vi "Create NI-DCPower Sessio.vi"(8 "error in (no error)":errorcluster, 10 "session information":T3, 11 "gRPC channel pool":T1) -> (0 "error out":errorcluster, 2 "instrument handle":refnum<k15>, 3 "gRPC channel pool out":T1)   [LabVIEW 2020, in "NIDCPowerSourceDCVoltage.lvlib"]
doc: "Creates and returns an gRPC based NI DC power instrument handle."
uses:
  NIDCPowerSourceDCVoltage.lvlib
  <vilib>/MeasurementLink/MeasurementLink Session Management Client/RPC Messages/ni_measurementlink_sessionmanagement_v1_SessionInformation.ctl
  <vilib>/MeasurementLink/MeasurementLink Session Management Client/RPC Messages/nidevice_grpc_Session.ctl
  <vilib>/MeasurementLink/MeasurementLink Session Management Client/RPC Messages/ni_measurementlink_sessionmanagement_v1_ChannelMapping.ctl
  GRPC Clients.ctl
  <vilib>/gRPC/LabVIEW gRPC Library/Shared/grpcId.ctl
  <vilib>/MeasurementLink/MeasurementLink Session Management Client/MeasurementLink Session Management Client.lvlib
  <vilib>/gRPC/LabVIEW gRPC Library/grpc-lvsupport-release.lvlib
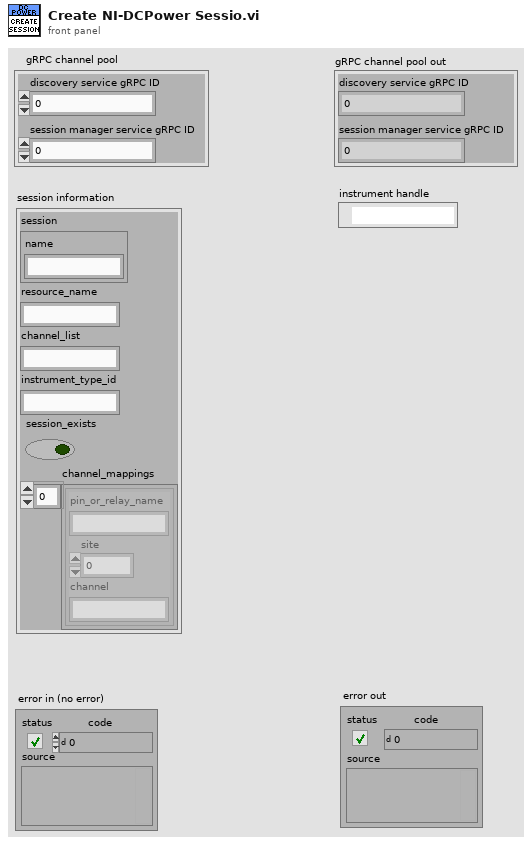
[diagram p1: front panel]
types:
  T1 = typedef "NIDCPowerSourceDCVoltage.lvlib/GRPC Clients.ctl" = cluster{"discovery service gRPC ID":T2, "session manager service gRPC ID":T2}
  T2 = typedef "grpc-lvsupport-release.lvlib/grpcId.ctl" = u64
  T3 = typedef "MeasurementLink Session Management Client.lvlib/ni_measurementlink_sessionmanagement_v1_SessionInformation.ctl" = cluster{"session":T4, "resource_name":string, "channel_list":string, "instrument_type_id":string, "session_exists":bool, "channel_mappings":T5[]}
  T4 = typedef "MeasurementLink Session Management Client.lvlib/nidevice_grpc_Session.ctl" = cluster{"name":string}
  T5 = typedef "MeasurementLink Session Management Client.lvlib/ni_measurementlink_sessionmanagement_v1_ChannelMapping.ctl" = cluster{"pin_or_relay_name":string, "site":i32, "channel":string}
  T6 = typedef "MeasurementLink Discovery Client.lvlib/ni_measurementlink_discovery_v1_ServiceLocation.ctl" = cluster{"location":string, "insecure_port":string, "ssl_authenticated_port":string}
  T7 = typedef "niDCPower gRPC Device Server.ctl" = cluster{"session name":string, "address (localhost)":string, "port (31763)":u32}
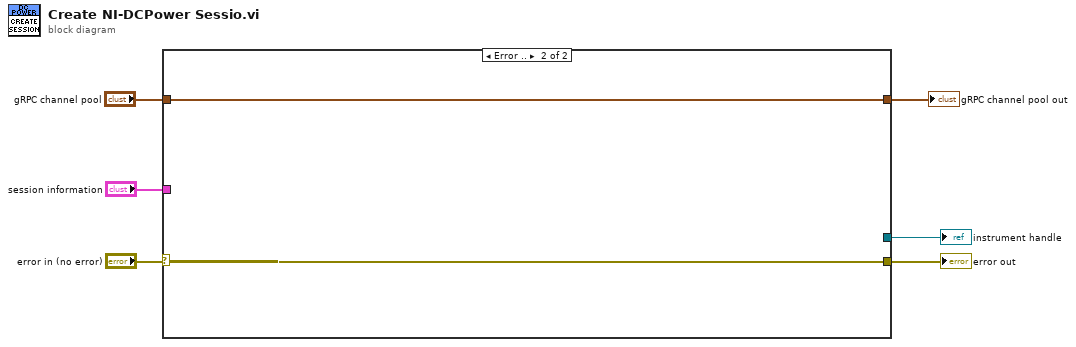
[diagram p0: block diagram]
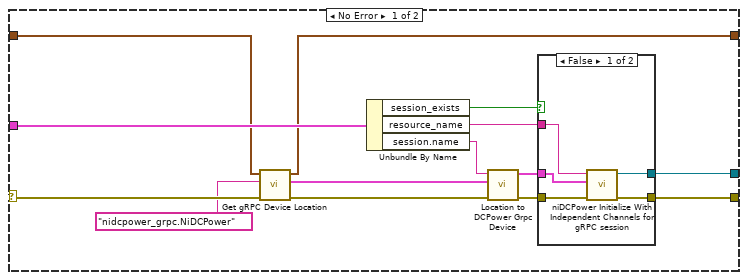
[diagram p2: hidden frame]
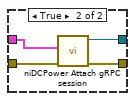
[diagram p3: hidden frame]
diagram:
  n1 = case shown="Error .." "error in (no error)" {
    selector: "error in (no error)" -> [w12 w30]
    tunnel: "session information" -> [w19 _]
    tunnel: [w14 w30] -> w5
    tunnel: [w13 _] -> w4
    tunnel: "gRPC channel pool" -> [w10 w29]
    tunnel: [w7 w29] -> w1
    frame No Error {
      n2 = call "Get gRPC Device Location.vi"("error in"=w12, "provided_interface"="nidcpower_grpc.NiDCPower", "gRPC channel pool"=w10) -> ("error out"=w11:errorcluster, "gRPC device location"=w8:T6, "gRPC channel pool out"=w7:T1)  [unwired: 6 in]
      n3 = Unbundle By Name(w19) -> ("session_exists"=w18:bool, "resource_name"=w15:string, "session.name"=w17:string)
      n4 = call "Location to DCPower Grpc Device.vi"("Grpc Device Location"=w8, "Session Name"=w17) -> ("NI gRPC Device Server Out"=w16:T7)  [unwired: 9 in]
      n5 = case shown="False" w18 {
        tunnel: w16 -> [w22 w26]
        tunnel: w15 -> [w21 _]
        tunnel: w11 -> [w24 w28]
        tunnel: [w23 w27] -> w14
        tunnel: [w20 w25] -> w13
        frame False {
          n6 = call <instrlib>:"niDCPower Initialize With Independent Channels for gRPC session.vi"("error in (no error)"=w24, "gRPC options"=w22, "resource name"=w21) -> ("error out"=w23:errorcluster, "instrument handle out"=w20:refnum<k15>)  [unwired: 7 in]
        }
        frame True {
          n7 = call <instrlib>:"niDCPower Attach gRPC session.vi"("error in (no error)"=w28, "gRPC options"=w26) -> ("error out"=w27:errorcluster, "instrument handle out"=w25:refnum<k15>)  [unwired: 8 in]
        }
      }
    }
    frame Error {
    }
  }
  "instrument handle" <- w4
  "error out" <- w5
  "gRPC channel pool out" <- w1
